vi "analyseData.vi"(8 "error in (no error)":errorcluster, 10 "HGF_VariantDataObject in":refnum<class "HGF_VariantDataObject.lvclass">, 11 "Wfm_PulseMeasurement in":refnum<class "Wfm_PulseMeasurement.lvclass">) -> (0 "error out":errorcluster, 2 "HGF_VariantDataObject out":refnum<class "HGF_VariantDataObject.lvclass">, 3 "Wfm_PulseMeasurement out":refnum<class "Wfm_PulseMeasurement.lvclass">)   [LabVIEW 2012, in "MyApp.lvlib" / "Wfm_PulseMeasurement.lvclass"]
doc: "Analyse data contained in HGF_DataVariantObject by using the HGF_DataAnalysator objects and optionally compining their results for a summaray result.\n\nThis is a dynamic dispatch VI to be overwritten by child classes."
uses:
  Wfm_PulseMeasurement.lvclass
  HGF_LVC/HGF_BaseClasses/HGF_VariantDataObject/HGF_VariantDataObject.lvclass
  Wfm_PulseMeasurement.lvclass/Wfm_PulseMeasurement.ctl
  <vilib>/measure/mascope.llb/Pulse Measurements 1 chan.vi
  <vilib>/measure/NI_MAPro.lvlib
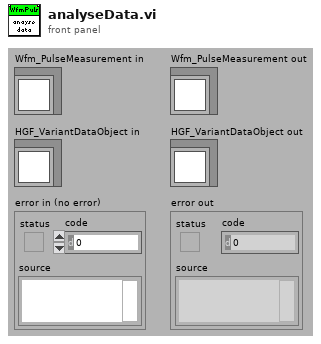
[diagram p1: front panel]
types:
  T1 = cluster{"pulse center":dbl, "ref levels":cluster{"high ref level":dbl, "mid ref level":dbl, "low ref level":dbl, "ref units":u16}}
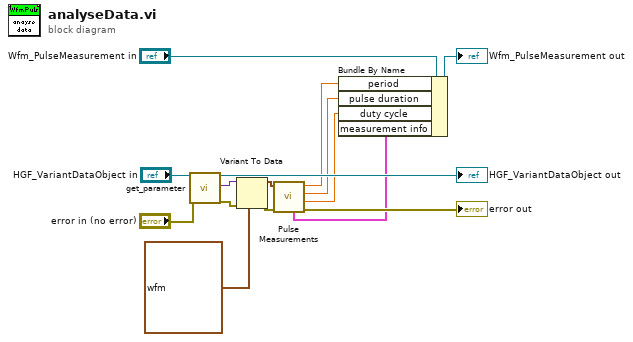
[diagram p0: block diagram]
diagram:
  n1 = call "get_parameter.vi"("HGF_VariantDataObject"="HGF_VariantDataObject in", "error in (no error)"="error in (no error)") -> ("dup HGF_VariantDataObject"=→"HGF_VariantDataObject out":refnum<class "HGF_VariantDataObject.lvclass">, "parameter"=w12:variant, "error out"=w10:errorcluster)  [unwired: 14 in, 1 out]
  n2 = Variant To Data(error in=w10, type=waveform(dbl) {"t0"=timestamp(0 s since 1904-01-01), "dt"=1.0, "Y"=[]} ("signal in"), Variant=w12) -> (data=w7:waveform(dbl), error out=w6:errorcluster)
  n3 = call-poly <vilib>:"Pulse Measurements.vi"("error in (no error)"=w6, "signal in"=w7) -> ("error out"=→"error out":errorcluster, "duty cycle"=w3:dbl, "pulse duration"=w4:dbl, "period"=w5:dbl, "measurement info"=w1:T1)  [unwired: 5 in]
  n4 = Bundle By Name(cluster="Wfm_PulseMeasurement in", "period"=w5, "pulse duration"=w4, "duty cycle"=w3, "measurement info"=w1) -> (→"Wfm_PulseMeasurement out":refnum<class "Wfm_PulseMeasurement.lvclass">)
